vi "refresh.vi"(8 "error in (no error)":errorcluster, 11 "window in":refnum<class "rywindow.lvclass">) -> (0 "error out":errorcluster, 3 "window out":refnum<class "rywindow.lvclass">)   [LabVIEW 2017, in "rywindow.lvclass"]
uses:
  rywindow.lvclass
  <vilib>/Utility/miscctls.llb/LVRowAndColumnTypeDef.ctl
  rywindow.lvclass/rywindow.ctl
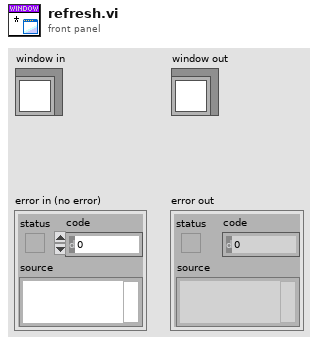
[diagram p1: front panel]
types:
  T1 = typedef "LVRowAndColumnTypeDef.ctl" = cluster{"Row":i32, "Column":i32}
  T2 = typedef "rywindow.lvclass/data.ctl" = cluster{"threads":T3[], "MinSize":cluster{"Width":u32, "Height":u32}, "font":T4, "active":i32}
  T3 = typedef "rywindow.lvclass/thread.ctl" = cluster{"name":string, "vi":refnum<vi>}
  T4 = typedef "LVFontTypeDef.ctl" = cluster{"Font Name":string, "Size":u16, "Bold":bool, "Italic":bool, "Underline":bool, "Strikeout":bool, "Color":u32}
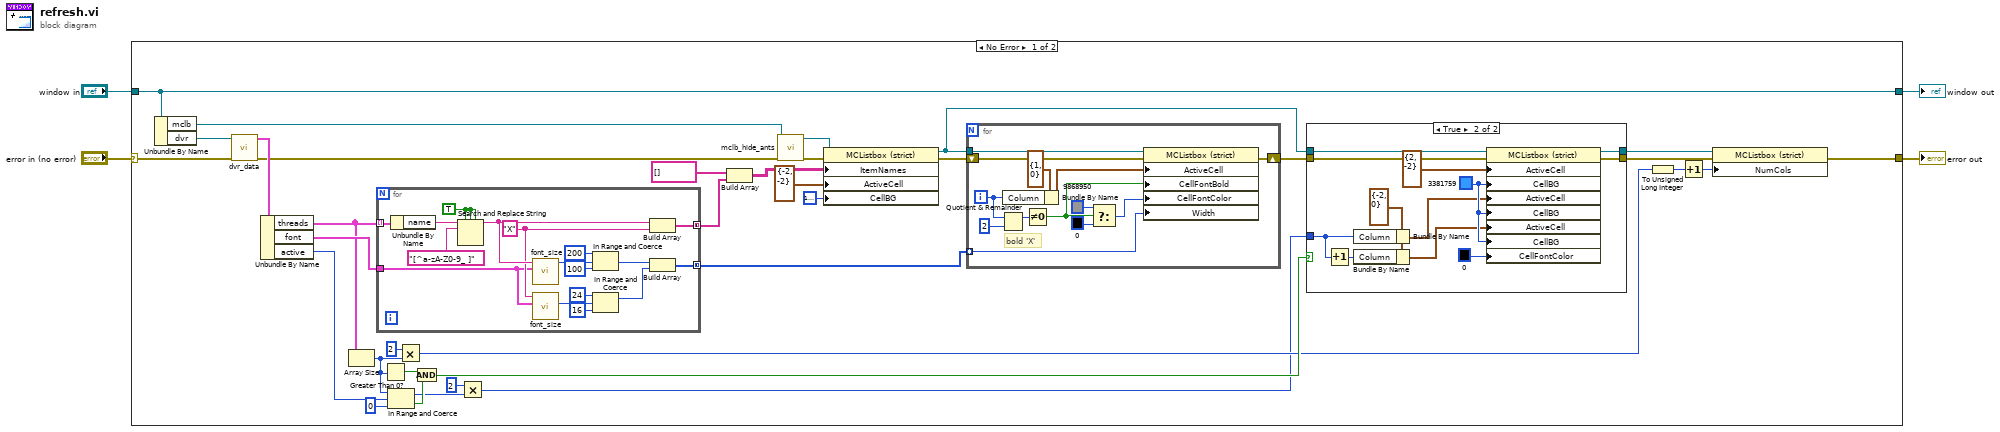
[diagram p0: block diagram]
diagram:
  n1 = case shown="No Error" "error in (no error)" {
    selector: "error in (no error)" -> [w38 w85]
    tunnel: [w9 w85] -> w3
    tunnel: [w39 w84] -> w1
    tunnel: "window in" -> [w39 w84]
    frame No Error {
      n2 = Unbundle By Name(w39) -> ("mclb"=w6:refnum<vi>, "dvr"=w37:refnum<data-value>)
      n3 = call "dvr_data.vi"("error in (no error)"=w38, "dvr"=w37) -> ("error out"=w8:errorcluster, "data"=w32:T2)  [unwired: 8 in]
      n4 = Unbundle By Name(w32) -> ("threads"=w34:T3[], "font"=w36:T4, "active"=w35:i32)
      n5 = Array Size(array=w34) -> (size(s)=w14:i32)
      n6 = for {
        tunnel: w34 -> [w83] mode=indexing
        tunnel: w36 -> [w77]
        tunnel: [w75] -> w31 mode=concatenating
        tunnel: [w74] -> w19 mode=concatenating
        w78 = "X" ("element")
        w80 = TRUE ("replace all? (F)")
        n7 = Unbundle By Name(w83) -> ("name"=w82:string)
        n8 = Search and Replace String(replace all?=w80, case sensitive?=w80, multiline?=w80, input string=w82, search string="[^a-zA-Z0-9_ ]") -> (result string=w79:string)  [unwired: 3 in, 3 out]
        n9 = call "font_size.vi"("cell font"=w77, "text"=w79) -> ("width"=w76:u32)  [unwired: 8 in, 1 out]
        n10 = call "font_size.vi"("cell font"=w77, "text"=w78) -> ("height"=w68:u32)  [unwired: 8 in, 1 out]
        n11 = In Range and Coerce(upper limit=u32 200, x=w76, lower limit=u32 100) -> (coerced(x)=w73:u32)  [unwired: 1 out]
        n12 = In Range and Coerce(upper limit=u32 24, x=w68, lower limit=u32 16) -> (coerced(x)=w67:u32)  [unwired: 1 out]
        n13 = Build Array(w79, w78) -> (w75:string[])
        n14 = Build Array(w73, w67) -> (w74:u32[])
      }
      n15 = Greater Than 0?(x=w14) -> (x > 0?=w24:bool)
      n16 = In Range and Coerce(upper limit=w14, x=w35, lower limit=0) -> (coerced(x)=w17:i32, In Range?=w25:bool)
      n17 = Multiply(x=2 ("y"), y=w14) -> (x*y=w12:i32)
      n18 = And(x=w24, y=w25) -> (x .and. y?=w23:bool)
      n19 = Multiply(x=2, y=w17) -> (x*y=w11:i32)
      n20 = Build Array(string[] [] ("element"), w31) -> (w29:string[][])
      n21 = call "mclb_hide_ants.vi"("error in (no error)"=w8, "mclb in"=w6) -> ("error out"=w7:errorcluster, "mclb out"=w5:refnum<vi>)  [unwired: 8 in]
      n22 = property class="MCListbox (strict)"(reference=w5, error in=w7, "ItemNames"=w29, "ActiveCell"=T1 {"Row"=-2, "Column"=-2} ("Active Cell:Active Cell"), "CellBG"=u32 16777216) -> (reference out=w20:refnum<vi>, error out=w22:errorcluster)
      n23 = for {
        tunnel: w20 -> [w63]
        shift-right: [w65] -> w21
        shift-left: w22 -> [w66]
        tunnel: w19 -> [w62] mode=indexing
        i -> [w60]
        # "bold 'X'"
        n24 = Quotient & Remainder(x=w60, y=2) -> (x-y*floor(x/y)=w58:i32)  [unwired: 1 out]
        n25 = Bundle By Name(cluster=T1 {"Row"=1, "Column"=0} ("Active Cell:Active Cell"), "Column"=w60) -> (w61:T1)
        n26 = Not Equal To 0?(x=w58) -> (x != 0?=w57:bool)
        n27 = Select(t=u32 9868950, s=w57, f=u32 0) -> (s? t:f=w54:u32)
        n28 = property class="MCListbox (strict)"(reference=w63, error in=w66, "ActiveCell"=w61, "CellFontBold"=w57, "CellFontColor"=w54, "Width"=w62) -> (error out=w65:errorcluster)  [unwired: 1 out]
      }
      n29 = case shown="True" w23 {
        tunnel: w21 -> [w41 w53]
        tunnel: [w41 w52] -> w26
        tunnel: w20 -> [w40 w51]
        tunnel: w11 -> [_ w47]
        tunnel: [w40 w48] -> w16
        frame False {
        }
        frame True {
          w49 = u32 3381759
          w50 = T1 {"Row"=-2, "Column"=0} ("Active Cell:Active Cell")
          n30 = Increment(x=w47) -> (x+1=w46:i32)
          n31 = Bundle By Name(cluster=w50, "Column"=w47) -> (w44:T1)
          n32 = Bundle By Name(cluster=w50, "Column"=w46) -> (w43:T1)
          n33 = property class="MCListbox (strict)"(reference=w51, error in=w53, "ActiveCell"=T1 {"Row"=2, "Column"=-2} ("Active Cell:Active Cell"), "CellBG"=w49, "ActiveCell"=w44, "CellBG"=w49, "ActiveCell"=w43, "CellBG"=w49, "CellFontColor"=u32 0) -> (reference out=w48:refnum<vi>, error out=w52:errorcluster)
        }
      }
      n34 = To Unsigned Long Integer(number=w12) -> (unsigned 32bit integer=w15:u32)
      n35 = Increment(x=w15) -> (x+1=w10:u32)
      n36 = property class="MCListbox (strict)"(reference=w16, error in=w26, "NumCols"=w10) -> (error out=w9:errorcluster)  [unwired: 1 out]
    }
    frame Error {
    }
  }
  "error out" <- w3
  "window out" <- w1
